vi "Sub03_BilliardRect.vi"(8 "error in (no error)":errorcluster, 11 "appended path":path) -> (0 "error out":errorcluster, 3 "Billard rect":T1)   [LabVIEW 2019]
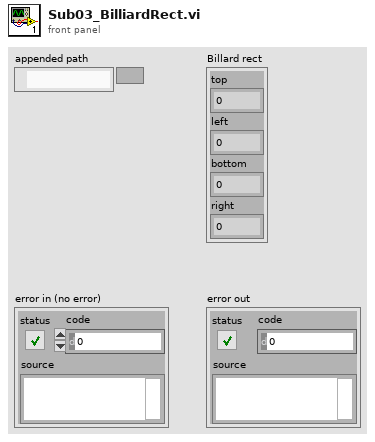
[diagram p1: front panel]
types:
  T1 = cluster{"top":dbl, "left":dbl, "bottom":dbl, "right":dbl}
  T2 = cluster{"left":u32, "top":u32, "right":u32, "bottom":u32}
  T3 = cluster{"R max":u32, "G max":u32, "B max":u32, "R min":u32, "G min":u32, "B min":u32}
  T4 = typedef "imagedata.ctl" = cluster{"image type":i32, "image depth":i32, "image":u8[], "mask":u8[], "colors":u32[], "Rectangle":cluster{"left":i16, "top":i16, "right":i16, "bottom":i16}}
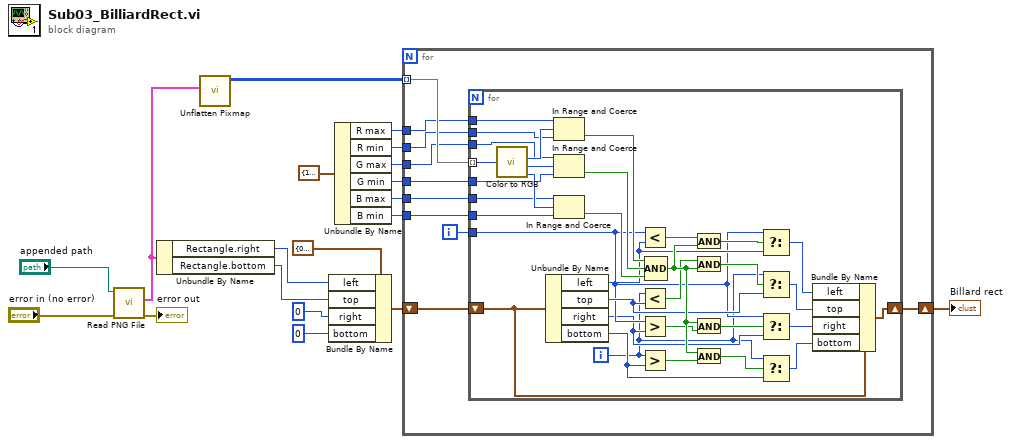
[diagram p0: block diagram]
diagram:
  n1 = call <vilib>:"Read PNG File.vi"("error in (no error)"="error in (no error)", "path to PNG file"="appended path") -> ("error out"=→"error out":errorcluster, "image data"=w7:T4)  [unwired: 7 in, 1 out]
  n2 = Unbundle By Name(w7) -> ("Rectangle.right"=w6:i16, "Rectangle.bottom"=w5:i16)
  n3 = call <vilib>:"Unflatten Pixmap.vi"("image data"=w7) -> ("24-bit pixmap"=w11:u32[][])  [unwired: 4 in, 6 out]
  n4 = Bundle By Name(cluster=T2 {"left"=0, "top"=0, "right"=0, "bottom"=0} ("Cluster"), "left"=w6, "top"=w5, "right"=u32 0, "bottom"=u32 0) -> (w3:T2)
  n5 = Unbundle By Name(T3 {"R max"=14, "G max"=42, "B max"=126, "R min"=0, "G min"=0, "B min"=121} ("Colors")) -> ("R max"=w13:u32, "R min"=w14:u32, "G max"=w15:u32, "G min"=w16:u32, "B max"=w17:u32, "B min"=w18:u32)
  n6 = for {
    tunnel: w11 -> [w29] mode=indexing
    tunnel: w13 -> [w28]
    tunnel: w14 -> [w27]
    tunnel: w15 -> [w26]
    tunnel: w16 -> [w25]
    tunnel: w17 -> [w24]
    tunnel: w18 -> [w23]
    shift-right: [w20] -> w19
    shift-left: w3 -> [w22]
    i -> [w21]
    n7 = for {
      tunnel: w29 -> [w63] mode=indexing
      tunnel: w28 -> [w59]
      tunnel: w27 -> [w58]
      tunnel: w26 -> [w57]
      tunnel: w25 -> [w56]
      tunnel: w24 -> [w55]
      tunnel: w23 -> [w54]
      tunnel: w21 -> [w35]
      shift-right: [w30] -> w20
      shift-left: w22 -> [w41]
      i -> [w31]
      n8 = call <vilib>:"Color to RGB.vi"("Color"=w63) -> ("R"=w62:u8, "G"=w61:u8, "B"=w60:u8)  [unwired: 1 out]
      n9 = Unbundle By Name(w41) -> ("left"=w39:u32, "top"=w37:u32, "right"=w34:u32, "bottom"=w32:u32)
      n10 = In Range and Coerce(upper limit=w59, x=w62, lower limit=w58) -> (In Range?=w53:bool)  [unwired: 1 out]
      n11 = In Range and Coerce(upper limit=w57, x=w61, lower limit=w56) -> (In Range?=w52:bool)  [unwired: 1 out]
      n12 = In Range and Coerce(upper limit=w55, x=w60, lower limit=w54) -> (In Range?=w51:bool)  [unwired: 1 out]
      n13 = Less?(x=w35, y=w39) -> (x < y?=w40:bool)
      n14 = Less?(x=w31, y=w37) -> (x < y?=w38:bool)
      n15 = Greater?(x=w35, y=w34) -> (0:w36:bool)
      n16 = Greater?(x=w31, y=w32) -> (0:w33:bool)
      n17 = Compound Arithmetic op=AND(w53, w52, w51) -> (w42:bool)
      n18 = And(x=w40, y=w42) -> (x .and. y?=w46:bool)
      n19 = And(x=w38, y=w42) -> (x .and. y?=w45:bool)
      n20 = And(x=w42, y=w36) -> (x .and. y?=w44:bool)
      n21 = And(x=w42, y=w33) -> (x .and. y?=w43:bool)
      n22 = Select(t=w35, s=w46, f=w39) -> (s? t:f=w50:u32)
      n23 = Select(t=w31, s=w45, f=w37) -> (s? t:f=w49:u32)
      n24 = Select(t=w35, s=w44, f=w34) -> (s? t:f=w48:u32)
      n25 = Select(t=w31, s=w43, f=w32) -> (s? t:f=w47:u32)
      n26 = Bundle By Name(cluster=w41, "left"=w50, "top"=w49, "right"=w48, "bottom"=w47) -> (w30:T2)
    }
  }
  "Billard rect" <- w19
